vi "PublicEvents.vi"(8 "error in (no error)":errorcluster, 10 "CurrentEvents":T1[](array[typedef]), 11 "SV_Publisher in":refnum<class "SV_Publisher.lvclass">) -> (0 "error out":errorcluster, 3 "SV_Publisher out":refnum<class "SV_Publisher.lvclass">)   [LabVIEW 2019, in "Logger.lvclass"]
uses:
  Logger.lvclass
  SV_Puplisher_class/SV_Publisher.lvclass
  EventData.ctl
  TypeDef/AlarmType.ctl
  Current Alarms.ctl
  SV_Puplisher_class/SV_Publisher.lvclass/SV_Publisher.ctl
  SV_Puplisher_class/Set SV.vi/1ae5d02c-efd0-450a-8aa4-8388e25d05bc.vi
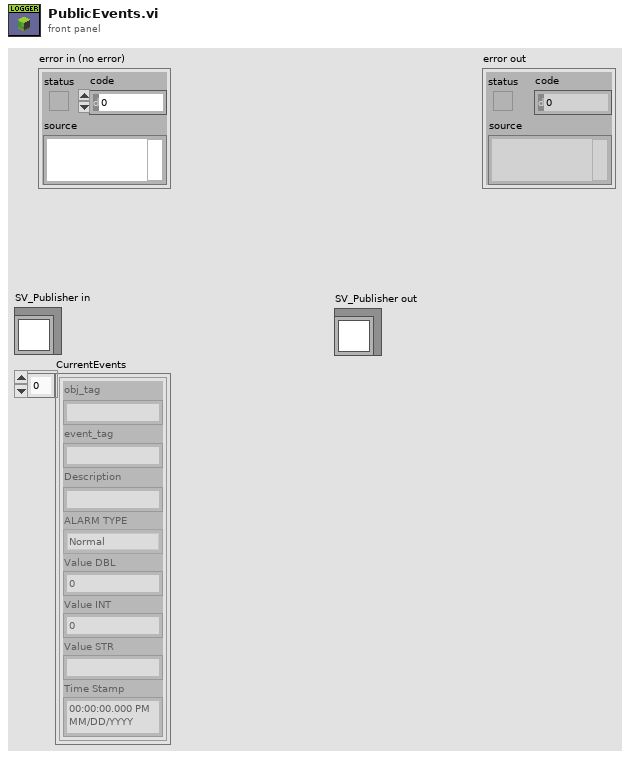
[diagram p1: front panel]
types:
  T1 = typedef "EventData.ctl" = cluster{"obj_tag":string, "event_tag":string, "Description":string, "ALARM TYPE":T2, "Value DBL":dbl, "Value INT":i32, "Value STR":string, "Time Stamp":timestamp}
  T2 = typedef "AlarmType.ctl" = enum16{"Normal", "Warning", "Alarm"}
  T3 = typedef "Current Alarms.ctl" = cluster{"alarms":T1[]}
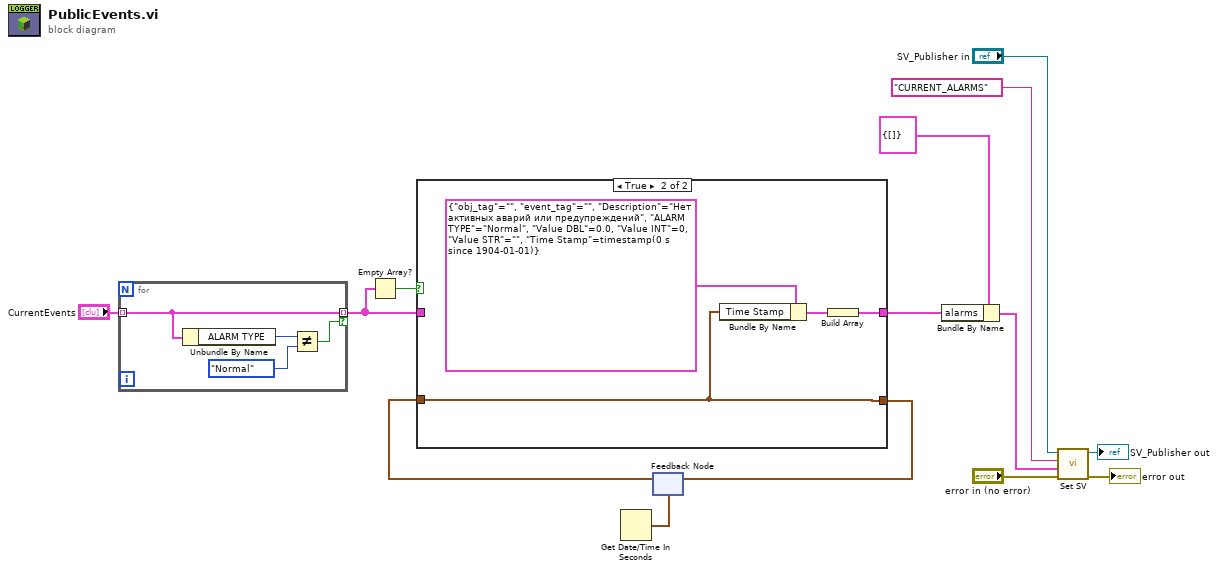
[diagram p0: block diagram]
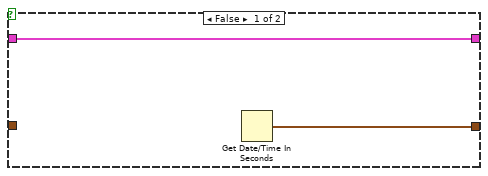
[diagram p2: hidden frame]
diagram:
  n1 = for {
    tunnel: "CurrentEvents" -> [w16] mode=indexing
    tunnel: [w16] -> w6 mode=indexing if=w15
    n2 = Unbundle By Name(w16) -> ("ALARM TYPE"=w18:T2)
    n3 = Not Equal?(x=w18, y=AlarmType."Normal") -> (x != y?=w15:bool)
  }
  n4 = Empty Array?(array=w6) -> (empty?=w8:bool)
  n5 = Get Date/Time In Seconds() -> (seconds since 1Jan1904=w1:timestamp)
  n6 = feedback #1(w1) -> (w2:timestamp)
  n7 = case shown="True" w8 {
    tunnel: [w20 w22] -> w7
    tunnel: w6 -> [w20 _]
    tunnel: [w19 w21] -> w3
    tunnel: w2 -> [_ w21]
    frame False {
      n8 = Get Date/Time In Seconds() -> (seconds since 1Jan1904=w19:timestamp)
    }
    frame True {
      n9 = Bundle By Name(cluster=T1 {"obj_tag"="", "event_tag"="", "Description"="Нет активных аварий или предупреждений", "ALARM TYPE"=enum."Normal", "Value DBL"=0.0, "Value INT"=0, "Value STR"="", "Time Stamp"=timestamp(0 s since 1904-01-01)} ("value"), "Time Stamp"=w21) -> (w23:T1)
      n10 = Build Array(w23) -> (w22:T1[])
    }
  }
  n11 = feedback-in #1(w3) -> ()
  n12 = Bundle By Name(cluster=T3 {"alarms"=[]} ("Current Alarms"), "alarms"=w7) -> (w14:T3)
  n13 = call "Set SV.vi"("error in (no error)"="error in (no error)", "SV Value"=w14, "SV Name"="CURRENT_ALARMS", "SV_Publisher in"="SV_Publisher in") -> ("error out"=→"error out":errorcluster, "SV_Publisher out"=→"SV_Publisher out":refnum<class "SV_Publisher.lvclass">)  [unwired: 6 in]
